vi "Export Section Database Change to CSV.vi"(9 "Database Changes":T1 {"Missing"."Node Ref" format="%.0x"; "Changed"."Old"."Node Ref" format="%.0x"}, 10 "Section":string, 11 "Folder":path) -> (0 "error out":errorcluster)   [LabVIEW 2025, in "Protection and Counter Addon System Explorer.lvlib"]
uses:
  Protection and Counter Addon System Explorer.lvlib
  Types/Database Changes.ctl
  Types/Base Frame Info_NoVS.ctl
  Types/Signal Attributes.ctl
  Types/CAN Filter Type.ctl
  Types/Base Frame Info.ctl
  <vilib>/NI VeriStand/Custom Device API/Custom Device Item Ref.ctl
  Types/Related CAN Frames.ctl
  Types/Related CAN Frames No VS.ctl
  <vilib>/Utility/error.llb/Trim Whitespace One-Sided.vi
  <vilib>/NI VeriStand/Custom Device API/Custom Device API.lvlib
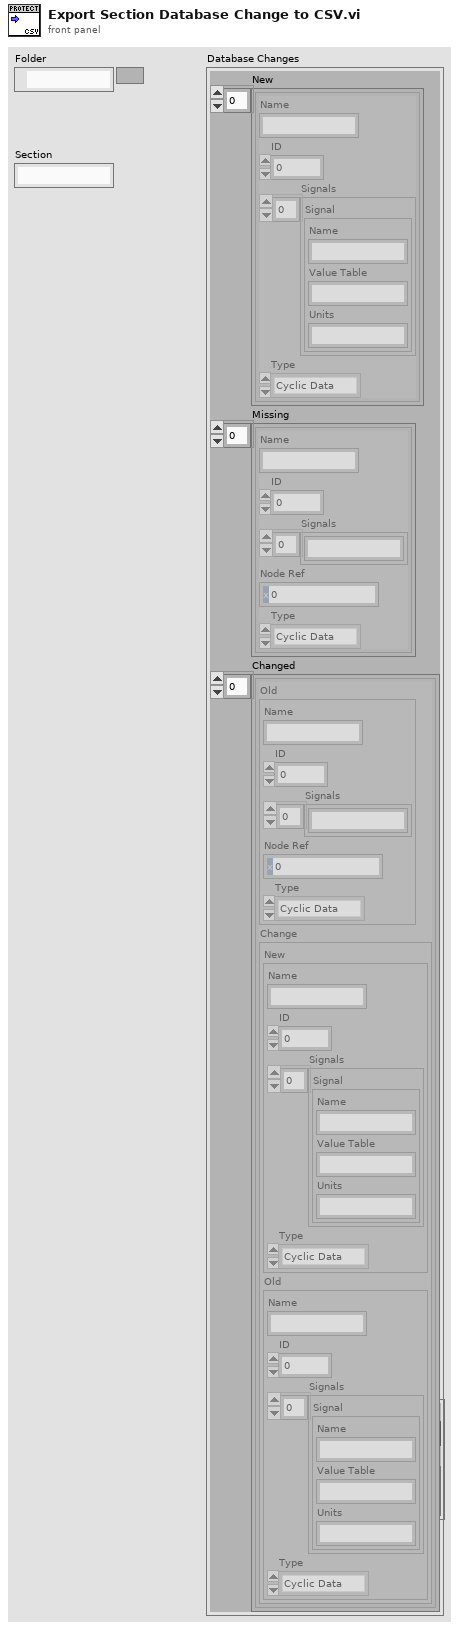
[diagram p1: front panel]
types:
  T1 = typedef "Protection and Counter Addon System Explorer.lvlib/Database Changes.ctl" = cluster{"New":T2[], "Missing":T5[], "Changed":T7[]}
  T2 = typedef "Protection and Counter Addon System Explorer.lvlib/Base Frame Info_NoVS.ctl" = cluster{"Name":string, "ID":u32, "Signals":T3[], "Type":T4}
  T3 = typedef "Protection and Counter Addon System Explorer.lvlib/Signal Attributes.ctl" = cluster{"Name":string, "Value Table":string, "Units":string}
  T4 = typedef "Protection and Counter Addon System Explorer.lvlib/CAN Filter Type.ctl" = enum16{"Cyclic Data", "Event Data", "Cyclic/Event", "All"}
  T5 = typedef "Protection and Counter Addon System Explorer.lvlib/Base Frame Info.ctl" = cluster{"Name":string, "ID":u32, "Signals":string[], "Node Ref":T6, "Type":T4}
  T6 = typedef "Custom Device API.lvlib/Custom Device Item Ref.ctl" = u64
  T7 = typedef "Protection and Counter Addon System Explorer.lvlib/Related CAN Frames.ctl" = cluster{"Old":T5, "Change":T8}
  T8 = typedef "Protection and Counter Addon System Explorer.lvlib/Related CAN Frames No VS.ctl" = cluster{"New":T2, "Old":T2}
  T9 = enum16{"open", "replace", "create", "open or create", "replace or create", "replace or create with confirmation"}
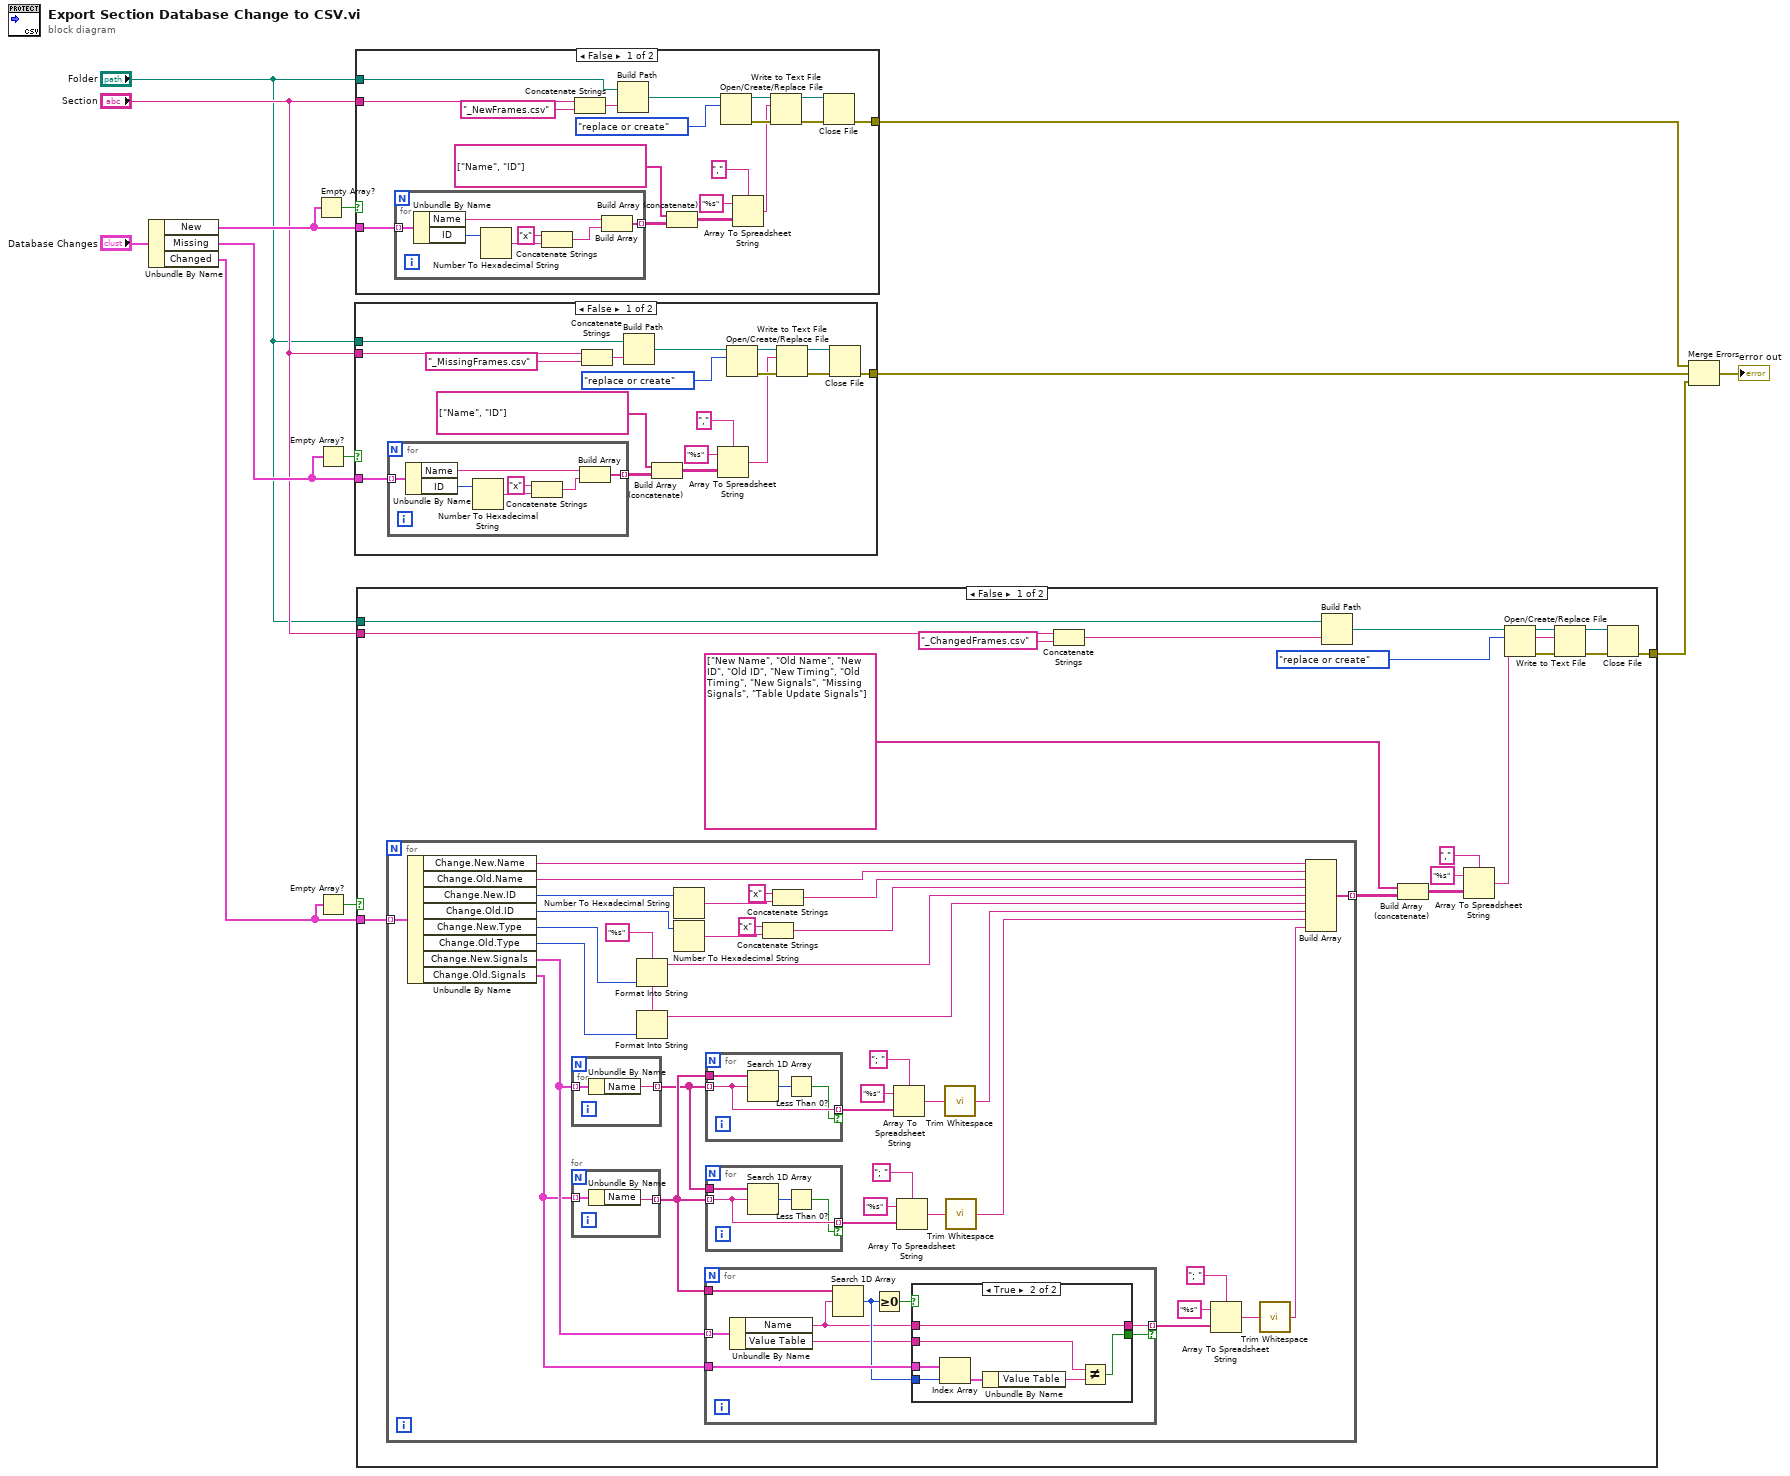
[diagram p0: block diagram]
diagram:
  n1 = Unbundle By Name("Database Changes") -> ("New"=w8:T2[], "Missing"=w11:T5[], "Changed"=w12:T7[])
  n2 = Empty Array?(array=w8) -> (empty?=w9:bool)
  n3 = Empty Array?(array=w11) -> (empty?=w10:bool)
  n4 = Empty Array?(array=w12) -> (empty?=w13:bool)
  n5 = case shown="False" w10 {
    tunnel: [w19 _] -> w3
    tunnel: "Folder" -> [w18 _]
    tunnel: "Section" -> [w15 _]
    tunnel: w11 -> [w14 _]
    frame False {
      n6 = for {
        tunnel: w14 -> [w38] mode=indexing
        tunnel: [w35] -> w28 mode=indexing
        n7 = Unbundle By Name(w38) -> ("Name"=w36:string, "ID"=w37:u32)
        n8 = Number To Hexadecimal String(2:w37) -> (0:w33:string)  [unwired: 1 in]
        n9 = Concatenate Strings("x" ("string"), w33) -> (w32:string)
        n10 = Build Array(w36, w32) -> (w35:string[])
      }
      n11 = Concatenate Strings(w15, "_MissingFrames.csv") -> (w16:string)
      n12 = Build Path(base path=w18, name or relative path=w16) -> (appended path=w20:path)
      n13 = Build Array (concatenate)(string[] ["Name", "ID"] ("appended array"), w28) -> (w31:string[][])
      n14 = Array To Spreadsheet String(delimiter (Tab)=",", array=w31, 3:"%s" ("format string")) -> (spreadsheet string=w21:string)
      n15 = Open/Create/Replace File(file path (use dialog)=w20, operation (0:open)=T9."replace or create") -> (refnum out=w25:refnum<file>, error out=w24:errorcluster)  [unwired: 4 in, 1 out]
      n16 = Write to Text File(file (use dialog)=w25, text=w21, error in=w24) -> (refnum out=w22:refnum<file>, error out=w23:errorcluster)  [unwired: 1 in, 1 out]
      n17 = Close File(refnum=w22, error in=w23) -> (error out=w19:errorcluster)  [unwired: 1 out]
    }
    frame True {
    }
  }
  n18 = case shown="False" w9 {
    tunnel: [w44 _] -> w2
    tunnel: "Folder" -> [w43 _]
    tunnel: "Section" -> [w40 _]
    tunnel: w8 -> [w39 _]
    frame False {
      n19 = for {
        tunnel: w39 -> [w63] mode=indexing
        tunnel: [w59] -> w53 mode=indexing
        n20 = Unbundle By Name(w63) -> ("Name"=w61:string, "ID"=w62:u32)
        n21 = Number To Hexadecimal String(2:w62) -> (0:w60:string)  [unwired: 1 in]
        n22 = Concatenate Strings("x" ("string"), w60) -> (w58:string)
        n23 = Build Array(w61, w58) -> (w59:string[])
      }
      n24 = Concatenate Strings(w40, "_NewFrames.csv") -> (w41:string)
      n25 = Build Path(base path=w43, name or relative path=w41) -> (appended path=w45:path)
      n26 = Build Array (concatenate)(string[] ["Name", "ID"] ("appended array"), w53) -> (w56:string[][])
      n27 = Open/Create/Replace File(file path (use dialog)=w45, operation (0:open)=T9."replace or create") -> (refnum out=w50:refnum<file>, error out=w49:errorcluster)  [unwired: 4 in, 1 out]
      n28 = Array To Spreadsheet String(delimiter (Tab)=",", array=w56, 3:"%s" ("format string")) -> (spreadsheet string=w46:string)
      n29 = Write to Text File(file (use dialog)=w50, text=w46, error in=w49) -> (refnum out=w47:refnum<file>, error out=w48:errorcluster)  [unwired: 1 in, 1 out]
      n30 = Close File(refnum=w47, error in=w48) -> (error out=w44:errorcluster)  [unwired: 1 out]
    }
    frame True {
    }
  }
  n31 = case shown="False" w13 {
    tunnel: w12 -> [w81 _]
    tunnel: [w68 _] -> w4
    tunnel: "Folder" -> [w67 _]
    tunnel: "Section" -> [w64 _]
    frame False {
      n32 = for {
        tunnel: w81 -> [w116] mode=indexing
        tunnel: [w112] -> w80 mode=indexing
        w99 = "%s" ("format string")
        n33 = Unbundle By Name(w116) -> ("Change.New.Name"=w117:string, "Change.Old.Name"=w114:string, "Change.New.ID"=w115:u32, "Change.Old.ID"=w113:u32, "Change.New.Type"=w100:T4, "Change.Old.Type"=w101:T4, "Change.New.Signals"=w94:T3[], "Change.Old.Signals"=w93:T3[])
        n34 = for {
          tunnel: w94 -> [w135] mode=indexing
          tunnel: [w134] -> w95 mode=indexing
          n35 = Unbundle By Name(w135) -> ("Name"=w134:string)
        }
        n36 = for {
          tunnel: w93 -> [w137] mode=indexing
          tunnel: [w136] -> w96 mode=indexing
          n37 = Unbundle By Name(w137) -> ("Name"=w136:string)
        }
        n38 = Format Into String(format string=w99, w100) -> (resulting string=w98:string)  [unwired: 2 in, 1 out]
        n39 = Format Into String(format string=w99, w101) -> (resulting string=w97:string)  [unwired: 2 in, 1 out]
        n40 = Number To Hexadecimal String(2:w115) -> (0:w85:string)  [unwired: 1 in]
        n41 = Number To Hexadecimal String(2:w113) -> (0:w83:string)  [unwired: 1 in]
        n42 = for {
          tunnel: w96 -> [w126]
          tunnel: w94 -> [w125] mode=indexing
          tunnel: w93 -> [w124]
          tunnel: [w120] -> w89 mode=indexing if=w118
          n43 = Unbundle By Name(w125) -> ("Name"=w119:string, "Value Table"=w121:string)
          n44 = Search 1D Array(1D array=w126, element=w119) -> (index of element=w123:i32)  [unwired: 1 in]
          n45 = Greater Or Equal To 0?(x=w123) -> (x >= 0?=w122:bool)
          n46 = case shown="True" w122 {
            tunnel: w124 -> [_ w133]
            tunnel: w123 -> [_ w132]
            tunnel: w121 -> [_ w129]
            tunnel: [_ w128] -> w120
            tunnel: w119 -> [_ w128]
            tunnel: [_ w127] -> w118
            frame False {
            }
            frame True {
              n47 = Index Array(array=w133, index=w132) -> (element=w131:T3)
              n48 = Unbundle By Name(w131) -> ("Value Table"=w130:string)
              n49 = Not Equal?(x=w129, y=w130) -> (x != y?=w127:bool)
            }
          }
        }
        n50 = for {
          tunnel: w96 -> [w141]
          tunnel: w95 -> [w139] mode=indexing
          tunnel: [w139] -> w107 mode=indexing if=w138
          n51 = Search 1D Array(1D array=w141, element=w139) -> (index of element=w140:i32)  [unwired: 1 in]
          n52 = Less Than 0?(x=w140) -> (x < 0?=w138:bool)
        }
        n53 = for {
          tunnel: w95 -> [w145]
          tunnel: w96 -> [w143] mode=indexing
          tunnel: [w143] -> w110 mode=indexing if=w142
          n54 = Search 1D Array(1D array=w145, element=w143) -> (index of element=w144:i32)  [unwired: 1 in]
          n55 = Less Than 0?(x=w144) -> (x < 0?=w142:bool)
        }
        n56 = Concatenate Strings("x" ("string"), w83) -> (w82:string)
        n57 = Concatenate Strings("x" ("string"), w85) -> (w84:string)
        n58 = Array To Spreadsheet String(delimiter (Tab)="; ", array=w107, 3:"%s" ("format string")) -> (spreadsheet string=w106:string)
        n59 = Array To Spreadsheet String(delimiter (Tab)="; ", array=w110, 3:"%s" ("format string")) -> (spreadsheet string=w111:string)
        n60 = call <vilib>:"Trim Whitespace.vi"("string"=w106) -> ("trimmed string"=w103:string)  [unwired: 1 in]
        n61 = call <vilib>:"Trim Whitespace.vi"("string"=w111) -> ("trimmed string"=w102:string)  [unwired: 1 in]
        n62 = Array To Spreadsheet String(delimiter (Tab)="; ", array=w89, 3:"%s" ("format string")) -> (spreadsheet string=w92:string)
        n63 = call <vilib>:"Trim Whitespace.vi"("string"=w92) -> ("trimmed string"=w88:string)  [unwired: 1 in]
        n64 = Build Array(w117, w114, w84, w82, w98, w97, w103, w102, w88) -> (w112:string[])
      }
      n65 = Concatenate Strings(w64, "_ChangedFrames.csv") -> (w65:string)
      n66 = Build Path(base path=w67, name or relative path=w65) -> (appended path=w69:path)
      n67 = Build Array (concatenate)(string[] ["New Name", "Old Name", "New ID", "Old ID", "New Timing", "Old Timing", "New Signals", "Missing Signals", "Table Update Signals"] ("appended array"), w80) -> (w78:string[][])
      n68 = Array To Spreadsheet String(delimiter (Tab)=",", array=w78, 3:"%s" ("format string")) -> (spreadsheet string=w70:string)
      n69 = Open/Create/Replace File(file path (use dialog)=w69, operation (0:open)=T9."replace or create") -> (refnum out=w74:refnum<file>, error out=w73:errorcluster)  [unwired: 4 in, 1 out]
      n70 = Write to Text File(file (use dialog)=w74, text=w70, error in=w73) -> (refnum out=w71:refnum<file>, error out=w72:errorcluster)  [unwired: 1 in, 1 out]
      n71 = Close File(refnum=w71, error in=w72) -> (error out=w68:errorcluster)  [unwired: 1 out]
    }
    frame True {
    }
  }
  n72 = Merge Errors(w2, w3, w4) -> (→"error out":errorcluster)
